vi "Salesforce OAuth Test.vi"() -> ()   [LabVIEW 2017]
uses:
  Oauth2/OAuth2 Flow -- enum.ctl
  Oauth2.Salesforce/Oauth2.Salesforce.lvclass/Oauth2.Salesforce.ctl
  Oauth2.Salesforce/Oauth2.Salesforce.lvclass
  D:/GitHub/Oauth2/source/Oauth2/Oauth2.lvclass
  Oauth2/Oauth2.lvclass
  <vilib>/LabVIEW Open Source Project/OpenURI/uri/URI.lvclass
  <vilib>/httpClient/LabVIEWHTTPClient.lvlib
panel:
  out "ID Token":T1
  out "issued_at":timestamp format="%^<%Y-%m-%dT%H:%M:%S%3uZ>T"
  out "Salesforce":string
  out "HTTP Response Headers":string
  in  "Consumer Secret":string="B8F58B0F0132D3DB9A2D1B4ECCB237D7B4BA4D3D03FF027ED4689F4597A8EFAE"
  in  "Consumer Key":string="3MVG9dAEux2v1sLtlchlC07icYhduQqXtXVDL6x4lz54Vkh_LM4FWFQz0AG0S4Mt5eo26phwX8RIn0unj8IYp"
  out "Salesforce Access Token":string
  out "error out":errorcluster
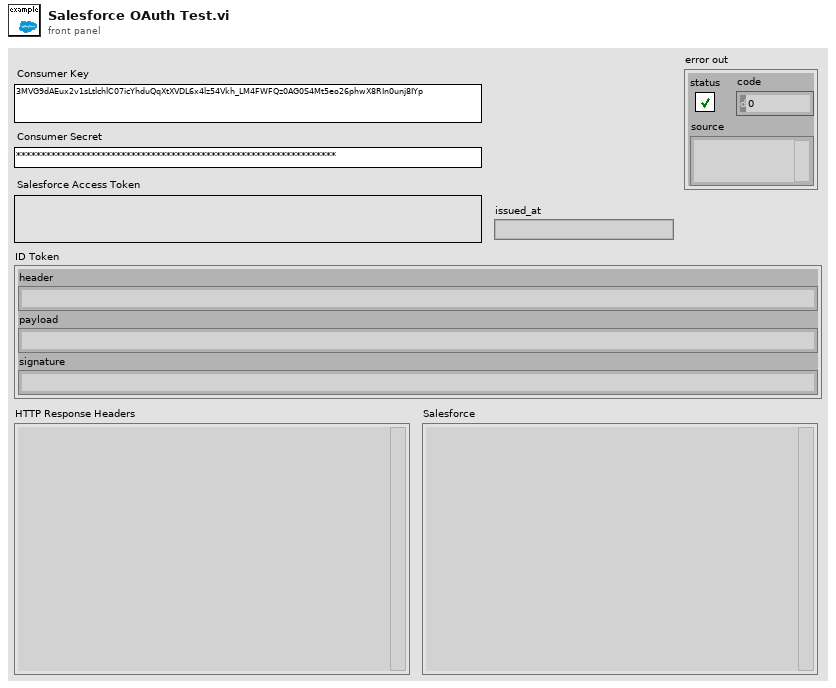
[diagram p1: front panel]
types:
  T1 = cluster{"header":string, "payload":string, "signature":string}
  T2 = typedef "Oauth2.lvclass/OAuth2 Flow -- enum.ctl" = enum16{"Authorization Code", "Authorization Code (PKCE)", "Implicit", "Resource Owner Credentials", "Client Credentials", "Refresh Token", "Device Code"}
  T3 = typedef "LabVIEWHTTPClient.lvlib/ClientHandle.ctl" = refnum<k1>
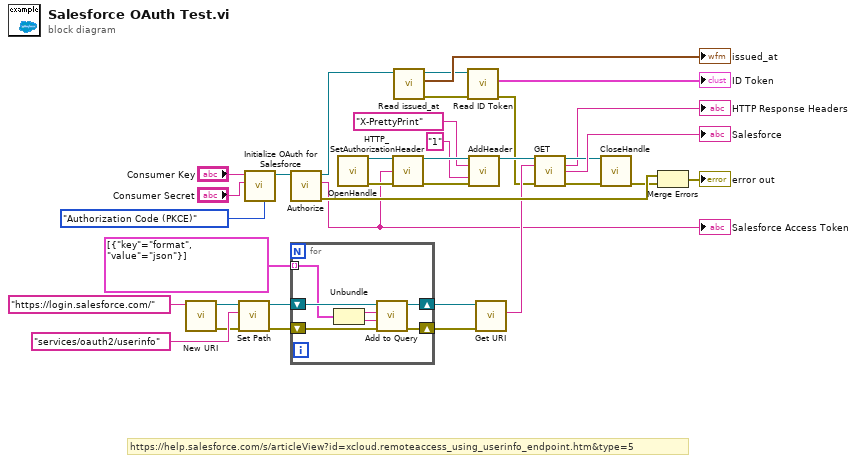
[diagram p0: block diagram]
diagram:
  # "https://help.salesforce.com/s/articleView?id=xcloud.remoteaccess_using_userinfo_endpoint.htm&type=5"
  n1 = call <vilib>:"New URI.vi"("URI"="https://login.salesforce.com/" ("path")) -> ("error out"=w24:errorcluster, "URI"=w35:refnum<class "URI.lvclass">)  [unwired: 9 in]
  n2 = call <vilib>:"Set Path.vi"("error in (no error)"=w24, "path"="services/oauth2/userinfo", "URI in"=w35) -> ("error out"=w22:errorcluster, "URI out"=w23:refnum<class "URI.lvclass">)  [unwired: 7 in]
  n3 = call "Initialize OAuth for Salesforce.vi"("Grant Flow (PKCE)"=OAuth2_Flow_--_enum."Authorization Code (PKCE)", "Client Secret"="Consumer Secret", "Client ID"="Consumer Key") -> ("Oauth2.Salesforce.lvclass"=w26:refnum<class "Oauth2.Salesforce.lvclass">)  [unwired: 7 in, 1 out]
  n4 = call "Authorize.vi"("Oauth2 in"=w26) -> ("error out"=w31:errorcluster, "Access Token"=w6:string, "Oauth2 out"=w12:refnum<class "Oauth2.Salesforce.lvclass">)  [unwired: 8 in]
  "Salesforce Access Token" <- w6
  n5 = for {
    shift-right: [w40] -> w21
    shift-left: w23 -> [w42]
    shift-right: [w39] -> w20
    shift-left: w22 -> [w41]
    tunnel: cluster{"key":string, "value":string}[] [{"key"="format", "value"="json"}] -> [w38] mode=indexing
    n6 = Unbundle(w38) -> ("key"=w37:string, "value"=w36:string)
    n7 = call <vilib>:"Add to Query.vi"("error in (no error)"=w41, "value"=w36, "key"=w37, "URI in"=w42) -> ("error out"=w39:errorcluster, "URI out"=w40:refnum<class "URI.lvclass">)  [unwired: 6 in]
  }
  n8 = call <vilib>:"OpenHandle.vi"() -> ("client handle out"=w33:T3, "error out"=w32:errorcluster)  [unwired: 14 in]
  n9 = call "HTTP_SetAuthorizationHeader.vi"("Client Handle"=w33, "Access Token"=w6, "error in (no error)"=w32) -> ("client handle dup"=w18:T3, "error out"=w17:errorcluster)  [unwired: 11 in]
  n10 = call "Read issued_at.vi"("Oauth2.Salesforce in"=w12) -> ("error out"=w9:errorcluster, "issued_at"=→"issued_at":timestamp, "Oauth2.Salesforce out"=w10:refnum<class "Oauth2.Salesforce.lvclass">)  [unwired: 8 in]
  n11 = call-dynamic "Read ID Token.vi"("error in (no error)"=w9, "Oauth2 in"=w10) -> ("error out"=w5:errorcluster, "ID Token"=→"ID Token":T1)  [unwired: 7 in, 1 out]
  n12 = call <vilib>:"AddHeader.vi"("client handle"=w18, "header"="X-PrettyPrint", "value"="1", "error in (no error)"=w17) -> ("client handle out"=w16:T3)  [unwired: 10 in, 1 out]
  n13 = call <vilib>:"Get URI.vi"("error in (no error)"=w20, "URI in"=w21) -> ("URI String"=w7:string)  [unwired: 7 in, 2 out]
  n14 = call <vilib>:"GET.vi"("client handle"=w16, "url"=w7, "error in (no error)"=w5) -> ("client handle out"=w3:T3, "headers"=→"HTTP Response Headers":string, "body"=→"Salesforce":string, "error out"=w4:errorcluster)  [unwired: 9 in]
  n15 = call <vilib>:"CloseHandle.vi"("client handle"=w3, "error in (no error)"=w4) -> ("error out"=w29:errorcluster)  [unwired: 13 in]
  n16 = Merge Errors(w31, w29) -> (→"error out":errorcluster)
